vi "AdminLogInColumnName(SubVI).vi"() -> (2 "Path for Score Table":string)   [LabVIEW 2013]
uses:
  FYP_LabviewGlobal(SubVI).vi
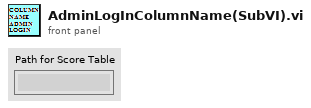
[diagram p1: front panel]
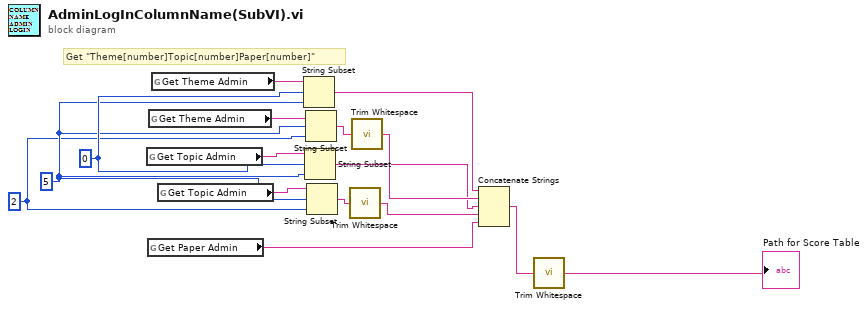
[diagram p0: block diagram]
diagram:
  w13 = 0
  w1 = 2
  w4 = 5
  # "Get \"Theme[number]Topic[number]Paper[number]\""
  n1 = global read "FYP_LabviewGlobal(SubVI).vi" "Get Topic Admin"() -> (w16:string)
  n2 = global read "FYP_LabviewGlobal(SubVI).vi" "Get Paper Admin"() -> (w2:string)
  n3 = global read "FYP_LabviewGlobal(SubVI).vi" "Get Theme Admin"() -> (w12:string)
  n4 = global read "FYP_LabviewGlobal(SubVI).vi" "Get Theme Admin"() -> (w15:string)
  n5 = global read "FYP_LabviewGlobal(SubVI).vi" "Get Topic Admin"() -> (w8:string)
  n6 = String Subset(string=w15, offset (0)=w13, length (rest)=w4) -> (substring=w10:string)
  n7 = String Subset(string=w16, offset (0)=w13, length (rest)=w4) -> (substring=w5:string)
  n8 = String Subset(string=w12, offset (0)=w4, length (rest)=w1) -> (substring=w11:string)
  n9 = String Subset(string=w8, offset (0)=w4, length (rest)=w1) -> (substring=w7:string)
  n10 = call <vilib>:"Trim Whitespace.vi"("string"=w7) -> ("trimmed string"=w6:string)  [unwired: 1 in]
  n11 = call <vilib>:"Trim Whitespace.vi"("string"=w11) -> ("trimmed string"=w9:string)  [unwired: 1 in]
  n12 = Concatenate Strings(w10, w9, w5, w6, w2) -> (w14:string)
  n13 = call <vilib>:"Trim Whitespace.vi"("string"=w14) -> ("trimmed string"=→"Path for Score Table":string)  [unwired: 1 in]
